vi "Teleop.vi"(10 "Match Info":T3={"Autonomous Elapsed Seconds"=0.0, "TeleOp Elapsed Seconds"=0.0, "Disabled Elapsed Seconds"=0.0, "Visited Autonomous"=FALSE, "Visited TeleOp"=FALSE, "Visited Disabled"=FALSE, "Autonomous Settings"={"Autonomous Style"=enum."Independent", "VI Refnum"=refnum}}, 11 "Call Context":T4) -> ()   [LabVIEW 2020]
doc: "This VI is called for each enabled TeleOp packet received from the DS. It is typically used to read from joysticks and other inputs and update I/O or setpoints for timed control loops. It should complete and return within 20 milliseconds or risk missing DS packets."
uses:
  <vilib>/Rock Robotics/WPI/DriverStation/WPI_DriverStationDerivedRobotMode.ctl
  <vilib>/Rock Robotics/WPI/DriverStation/WPI_DriverStationMatch Info.ctl
  Drive/Implementation/Robot Velocities.ctl
  Drive/Implementation/Driving Mode.ctl
  <vilib>/Rock Robotics/WPI/Joystick/XBox Buttons Indexer.ctl
  <vilib>/Rock Robotics/WPI/Joystick/XBox Axes Indexer.ctl
  97e635d3-2ee8-4cef-b098-8ad6758c7b24.vi
  <vilib>/Rock Robotics/WPI/Utilities/WPI_GetSetVariantRefNum.vi
panel:
  in  "Max Velocities":T1={"vx"=15.0, "vy"=15.0, "w"=270.0}
  in  "Deadband":dbl=0.1
  in  "Send Inputs":bool
  in  "Joystick Inputs":T2(array[cluster])
  in  "Simulated Teleop?":bool
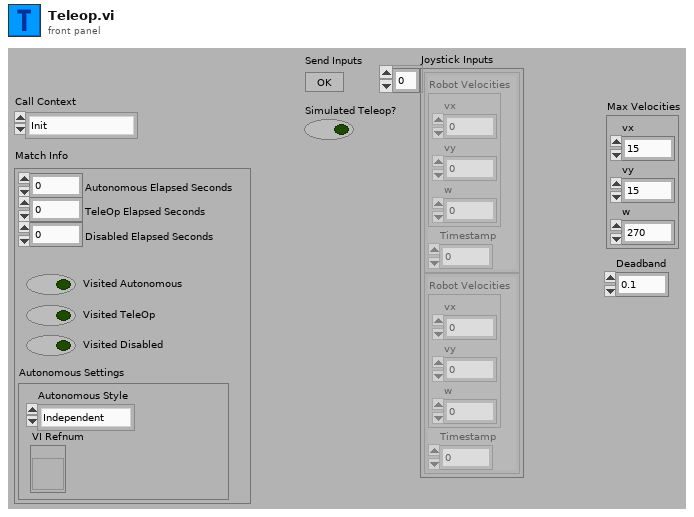
[diagram p1: front panel]
types:
  T1 = typedef "Robot Velocities.ctl" = cluster{"vx":dbl, "vy":dbl, "w":dbl}
  T2 = cluster{"Robot Velocities":T1, "Timestamp":dbl}[]
  T3 = typedef "WPI_DriverStationMatch Info.ctl" = cluster{"Autonomous Elapsed Seconds":dbl, "TeleOp Elapsed Seconds":dbl, "Disabled Elapsed Seconds":dbl, "Visited Autonomous":bool, "Visited TeleOp":bool, "Visited Disabled":bool, "Autonomous Settings":cluster{"Autonomous Style":enum16{"Iterative", "Independent"}, "VI Refnum":refnum<vi>}}
  T4 = typedef "WPI_DriverStationDerivedRobotMode.ctl" = enum16{"Init", "Execute", "Stop"}
  T5 = typedef "XBox Buttons Indexer.ctl" = enum16{"A", "B", "X", "Y", "Left Bumper", "Right Bumper", "Back", "Start", "Left Joystick", "Right Joystick"}
  T6 = typedef "Driving Mode.ctl" = enum16{"Robot Centric", "Field Centric"}
  T7 = typedef "WPI_JoystickDevRef.ctl" = cluster{"Device":T8}
  T8 = typedef "WPI_JoystickDeviceEnum.ctl" = enum16{"USB 0", "USB 1", "USB 2", "USB 3", "USB 4", "USB 5"}
  T9 = typedef "XBox Axes Indexer.ctl" = enum16{"Left X", "Left Y", "Left Trigger", "Right Trigger", "Right X", "Right Y"}
  T10 = typedef "CTRE_PigeonIMU_DeviceRef.ctl" = cluster{"DeviceStatus":errorcluster, "Device Number":u8, "Type":T11, "Device ID":u32, "Handle":u64, "UsageFrame":u32, "Library Path":path}
  T11 = typedef "CTRE_PigeonIMU_ConnectionType.ctl" = u32
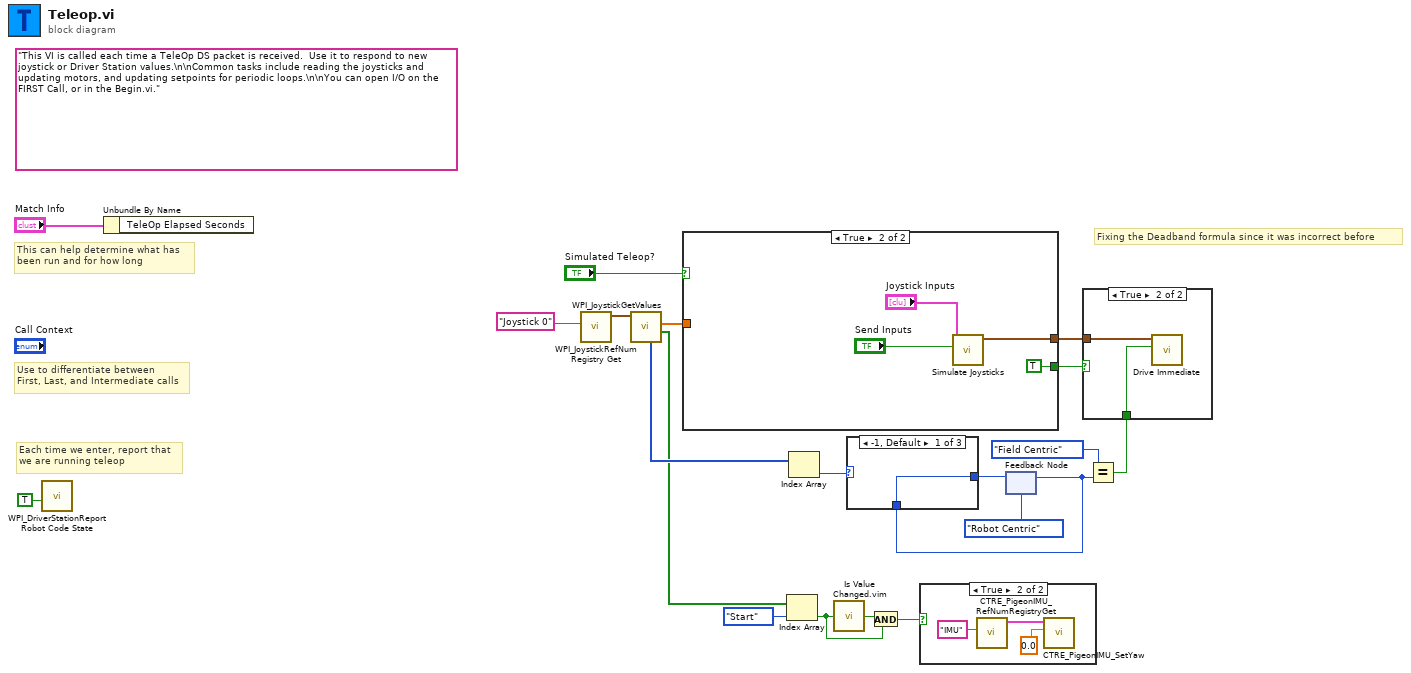
[diagram p0: block diagram]
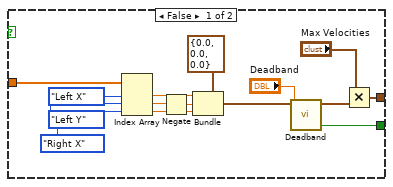
[diagram p2: hidden frame]
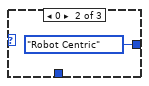
[diagram p4: hidden frame]
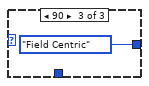
[diagram p5: hidden frame]
diagram:
  (unwired) "This VI is called each time a TeleOp DS packet is received.  Use it to respond to new joystick or Driver Station values.\n\nCommon tasks include reading the joysticks and updating motors, and updating setpoints for periodic loops.\n\nYou can open I/O on the FIRST Call, or in the Begin.vi."
  # "Fixing the Deadband formula since it was incorrect before"
  # "Each time we enter, report that\nwe are running teleop"
  # "Use to differentiate between\nFirst, Last, and Intermediate calls"
  # "This can help determine what has\nbeen run and for how long"
  n1 = call <vilib>:"WPI_DriverStationReport Robot Code State.vi"("TeleOp"=TRUE ("Autonomous")) -> ()  [unwired: 10 in, 1 out]
  n2 = Unbundle By Name("Match Info") -> ()  [unwired: 1 out]
  n3 = call <vilib>:"WPI_JoystickRefNum Registry Get.vi"("refnum name"="Joystick 0") -> ("JoystickDevRef"=w17:T7)  [unwired: 1 in, 9 out]
  n4 = call <vilib>:"WPI_JoystickGetValues.vi"("JoystickDevRef"=w17) -> ("Buttons"=w9:bool[], "Axes"=w16:dbl[], "POVs"=w14:i16[])  [unwired: 6 in, 2 out]
  n5 = case shown="True" "Simulated Teleop?" {
    tunnel: w16 -> [w35 _]
    tunnel: [w22 w39] -> w2
    tunnel: [w21 TRUE ("Sending Input?")] -> w1
    frame False {
      n6 = Index Array(array=w35, index #1=XBox_Axes_Indexer."Left X" ("XBox Axes"), index #2=XBox_Axes_Indexer."Left Y" ("XBox Axes"), index #3=XBox_Axes_Indexer."Right X" ("XBox Axes")) -> (element #1=w31:dbl, element #2=w28:dbl, element #3=w30:dbl)
      n7 = Negate(x=w28) -> (-x=w27:dbl)
      n8 = Bundle(cluster=T1 {"vx"=0.0, "vy"=0.0, "w"=0.0} ("Robot Velocities"), "vx"=w31, "vy"=w27, "w"=w30) -> (w23:T1)
      n9 = call "Deadband.vi"("Deadband"="Deadband", "Robot Velocities"=w23) -> ("Sending Input?"=w21:bool, "Adjusted Robot Velocities"=w25:T1)  [unwired: 8 in]
      n10 = Multiply(x="Max Velocities", y=w25) -> (x*y=w22:T1)
    }
    frame True {
      n11 = call "Simulate Joysticks.vi"("Send Inputs"="Send Inputs", "Joystick Inputs"="Joystick Inputs") -> ("Joystick Inputs"=w39:T1)  [unwired: 9 in]
    }
  }
  n12 = Index Array(array=w9, index=XBox_Buttons_Indexer."Start" ("XBox Buttons")) -> (element=w6:bool)
  n13 = Index Array(array=w14) -> (element=w13:i16)  [unwired: 1 in]
  n14 = call "Is Value Changed.vim"("value"=w6) -> ("changed or first call?"=w7:bool)
  n15 = And(x=w7, y=w6) -> (x .and. y?=w5:bool)
  n16 = case shown="True" w5 {
    frame False {
    }
    frame True {
      n17 = call <vilib>:"CTRE_PigeonIMU_RefNumRegistryGet.vi"("refnum name"="IMU") -> ("PigeonIMUDevRef"=w40:T10)  [unwired: 9 in, 1 out]
      n18 = call <vilib>:"CTRE_PigeonIMU_SetYaw.vi"("Value"=0.0, "PigeonIMUDevRef"=w40) -> ()  [unwired: 8 in, 2 out]
    }
  }
  n19 = feedback #1(Driving_Mode."Robot Centric") -> (w11:T6)
  n20 = case shown="-1, Default" w13 {
    tunnel: [w43 Driving_Mode."Robot Centric" Driving_Mode."Field Centric"] -> w12
    tunnel: w11 -> [w43 _ _]
    frame -1, Default {
    }
    frame 0 {
    }
    frame 90 {
    }
  }
  n21 = feedback-in #1(w12) -> ()
  n22 = Equal?(x=Driving_Mode."Field Centric", y=w11) -> (x = y?=w4:bool)
  n23 = case shown="True" w1 {
    tunnel: w4 -> [_ w47]
    tunnel: w2 -> [_ w46]
    frame False {
    }
    frame True {
      n24 = call "Drive Immediate.vi"("Field Centric?"=w47, "Robot Velocities"=w46) -> ()  [unwired: 9 in, 1 out]
    }
  }
